vi "SDO_DRIVE_BEGIN.vi"(8 "error in (no error)":errorcluster) -> (0 "error out":errorcluster, 2 "Gyro Reading":T1 {"SIN" format="%13.4f"; "COS" format="%13.4f"; "VALUE" format="%13.4f"}, 3 "SWERVE_DRIVE_KINEMATICS":T2 {"SavedModuleStates"."Angle"."SIN" format="%13.4f"; "SavedModuleStates"."Angle"."COS" format="%13.4f"; "SavedModuleStates"."Angle"."VALUE" format="%13.4f"; "PrevCoR"."Y" format="%14.3f"; "PrevCoR"."X" format="%14.3f"; "Modules"."Y" format="%14.3f"; "Modules"."X" format="%14.3f"})   [LabVIEW 2019]
uses:
  <vilib>/Rock Robotics/WPI/ThirdParty/JAS_Junk/TrajLib/TypeDef/SWERVE_DRIVE_KINEMATICS.ctl
  <vilib>/Analysis/Matrix/Datatypes/RealMatrix.ctl
  <vilib>/Rock Robotics/WPI/ThirdParty/JAS_Junk/TrajLib/TypeDef/TRANSLATION2D.ctl
  <vilib>/Rock Robotics/WPI/ThirdParty/JAS_Junk/TrajLib/TypeDef/SWERVE_DRIVE_MODULE_STATE.ctl
  <vilib>/Rock Robotics/WPI/ThirdParty/JAS_Junk/TrajLib/TypeDef/ROTATION2D.ctl
  <vilib>/Rock Robotics/SystemInterfaces/DIO/FPGA_DIOPWMChannel.ctl
  <vilib>/Rock Robotics/SystemInterfaces/DIO/FPGA_DIOChannel.ctl
  <vilib>/Rock Robotics/SystemInterfaces/AI/FPGA_AIGyroChannel.ctl
  <vilib>/Rock Robotics/WPI/ThirdParty/JAS_Junk/TrajLib/Conv_Deg_Radians.vi
  <vilib>/Rock Robotics/WPI/ThirdParty/JAS_Junk/TrajLib/Rotation2d_CreateAngle.vi
  <vilib>/Rock Robotics/WPI/ThirdParty/JAS_Junk/TrajLib/VI/BoolCmd_Send_Internal.vi
  <vilib>/Rock Robotics/WPI/ThirdParty/JAS_Junk/TrajLib/VI/BoolCmd_ObtainQueue.vi
  SDO_DRIVE_GLOBALS.vi
  <vilib>/Rock Robotics/WPI/ThirdParty/JAS_Junk/TrajLib/Trajectory_Library.lvlib
  <vilib>/Rock Robotics/SystemInterfaces/AI/FPGA_AIChannel.ctl
  <vilib>/Rock Robotics/SystemInterfaces/spilib/spi_bus.ctl
  <vilib>/Rock Robotics/WPI/Gyro/WPI_GyroDevRef.ctl
  <vilib>/Analysis/Matrix/NI_Matrix.lvlib
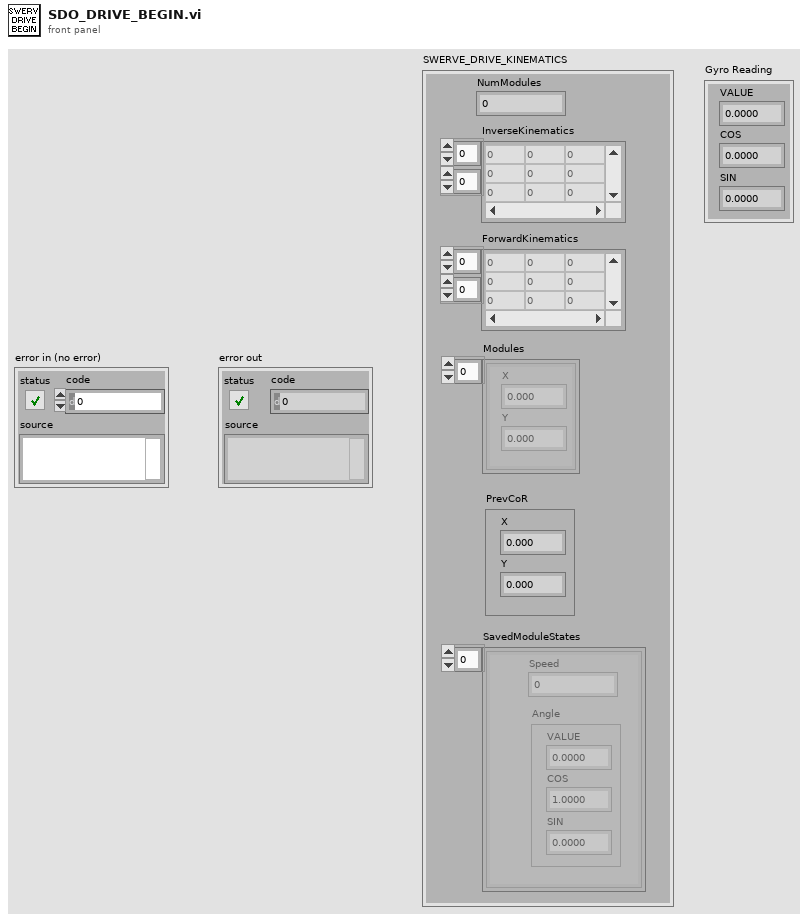
[diagram p1: front panel]
types:
  T1 = typedef "Trajectory_Library.lvlib/ROTATION2D.ctl" = cluster{"VALUE":dbl, "COS":dbl, "SIN":dbl}
  T2 = typedef "Trajectory_Library.lvlib/SWERVE_DRIVE_KINEMATICS.ctl" = cluster{"NumModules":i32, "InverseKinematics":T3, "ForwardKinematics":T3, "Modules":T4[], "PrevCoR":T4, "SavedModuleStates":T5[]}
  T3 = typedef "NI_Matrix.lvlib/RealMatrix.ctl" = dbl[][]
  T4 = typedef "Trajectory_Library.lvlib/TRANSLATION2D.ctl" = cluster{"X":dbl, "Y":dbl}
  T5 = typedef "Trajectory_Library.lvlib/SWERVE_DRIVE_MODULE_STATE.ctl" = cluster{"Speed":dbl, "Angle":T1}
  T6 = typedef "FPGA_AIGyroChannel.ctl" = enum8{"AI 0", "AI 1", "Invalid"}
  T7 = typedef "FPGA_DIOChannel.ctl" = enum8{"DIO 0", "DIO 1", "DIO 2", "DIO 3", "DIO 4", "DIO 5", "DIO 6", "DIO 7", "DIO 8", "DIO 9", "DIO MXP 0", "DIO MXP 1", "DIO MXP 2", "DIO MXP 3", "DIO MXP 4", "DIO MXP 5", "DIO MXP 6", "DIO MXP 7", "DIO MXP 8", "DIO MXP 9", "DIO MXP 10", "DIO MXP 11", "DIO MXP 12", "DIO MXP 13", "DIO MXP 14", "DIO MXP 15", "SPI Port CS1", "SPI Port CS2", "SPI Port CS3", "SPI Port MISO", "SPI Port MOSI", "Invalid"}
  T8 = typedef "FPGA_DIOPWMChannel.ctl" = enum8{"PWM 0", "PWM 1", "PWM 2", "PWM 3", "PWM 4", "PWM 5", "PWM 6", "PWM 7", "PWM 8", "PWM 9", "PWM MXP 0", "PWM MXP 1", "PWM MXP 2", "PWM MXP 3", "PWM MXP 4", "PWM MXP 5", "PWM MXP 6", "PWM MXP 7", "PWM MXP 8", "PWM MXP 9", "Invalid"}
  T9 = typedef "WPI_GyroDevRef.ctl" = cluster{"DevStatus":errorcluster, "Analog Channel":T10, "Gain (VoltsPerDegree/Second)":dbl, "Gyro Type":enum16{"Analog", "XRS450"}, "Handle":i32, "SPI Bus":T11, "Device Found":bool, "Sample Rate":dbl, "Calibrate On Open":bool, "Offset":dbl}
  T10 = typedef "FPGA_AIChannel.ctl" = enum8{"AI 0", "AI 1", "AI 2", "AI 3", "AI MXP 0", "AI MXP 1", "AI MXP 2", "AI MXP 3", "Invalid"}
  T11 = typedef "spi_bus.ctl" = enum16{"SPI On-Board, CS0", "SPI On-Board, CS1", "SPI On-Board, CS2", "SPI On-Board, CS3", "SPI MXP", "Invalid"}
  T12 = typedef "Trajectory_Library.lvlib/SWERVE_DRIVE_MODULE_POSITION.ctl" = cluster{"Distance":dbl, "Angle":T1, "P":bool}
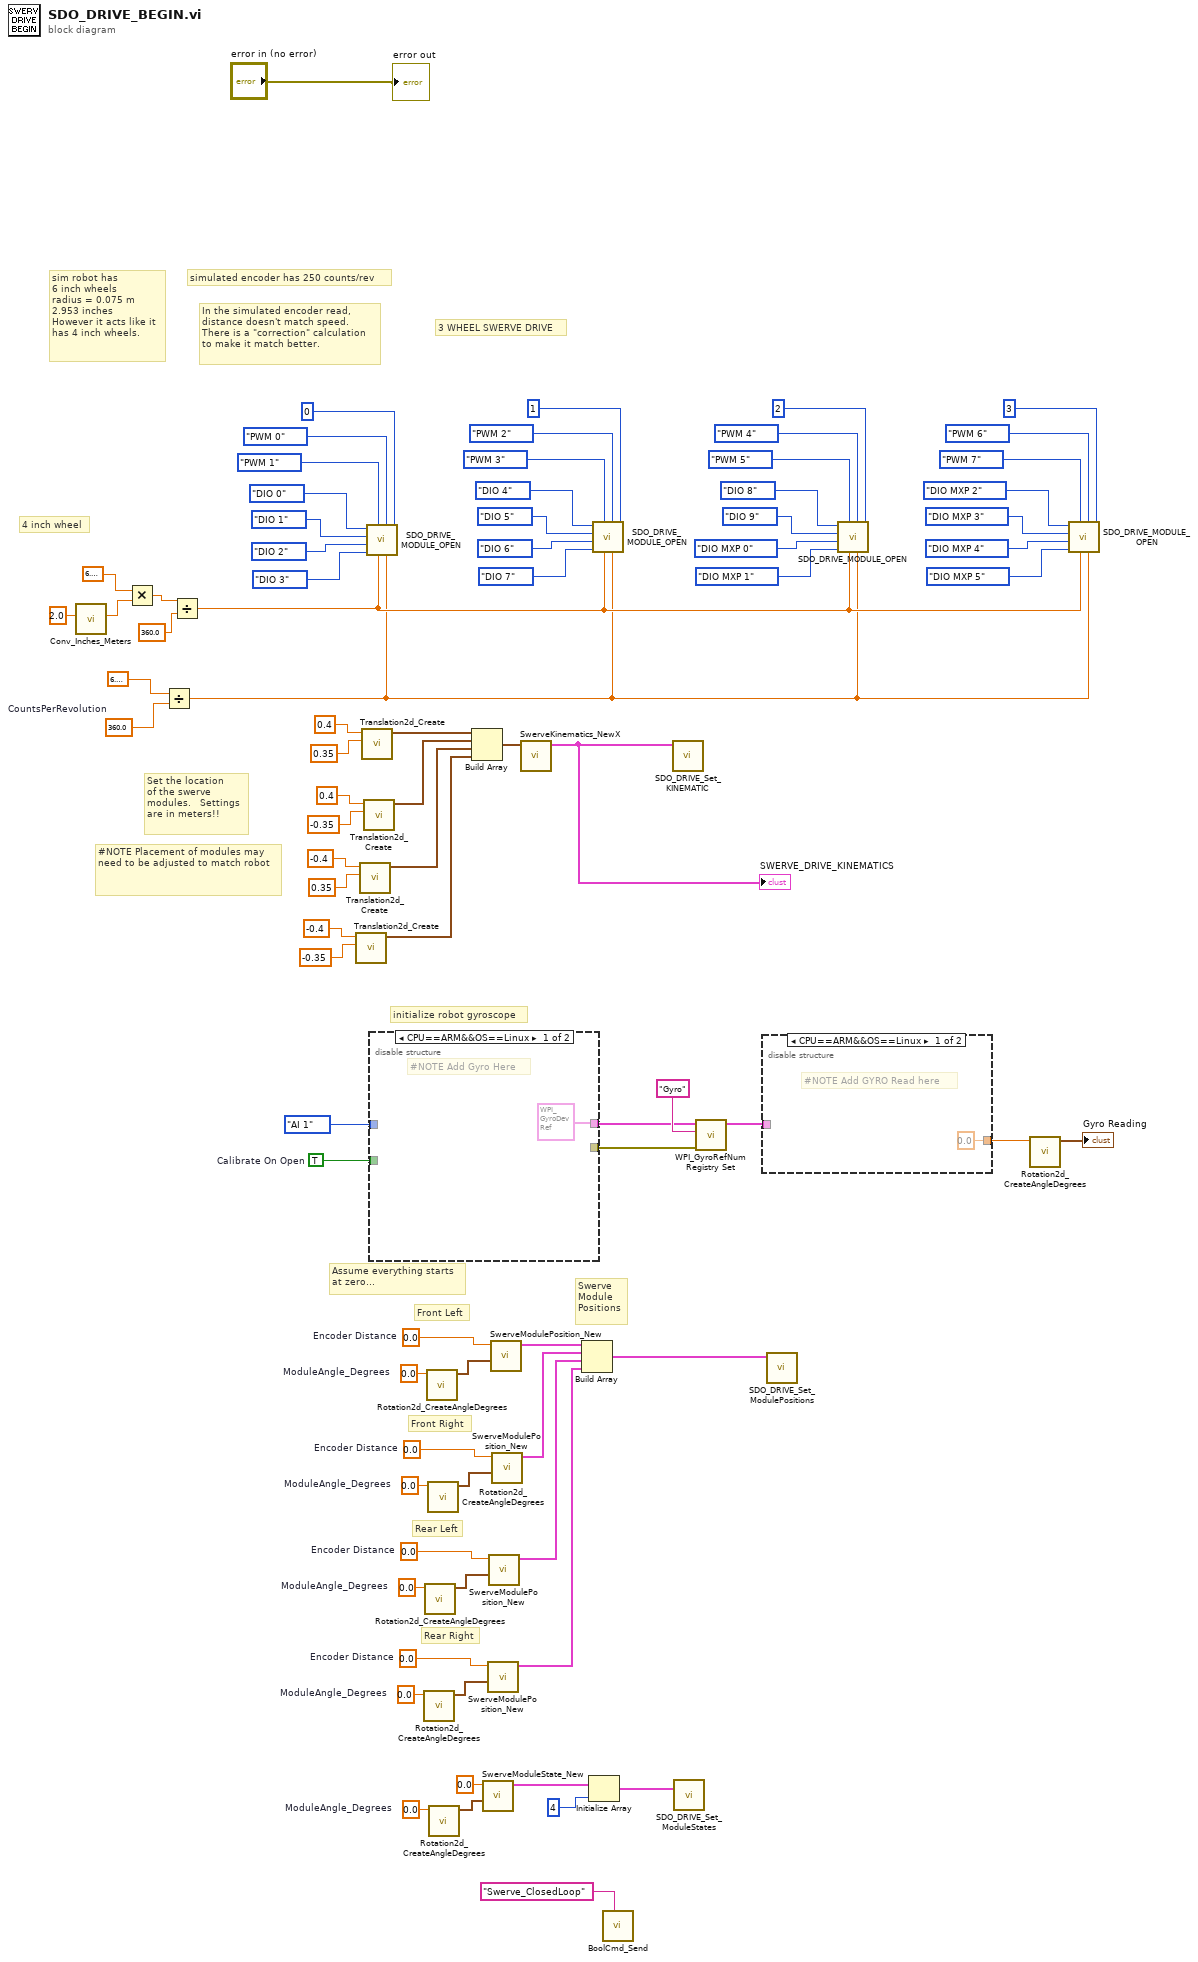
[diagram p0: block diagram]
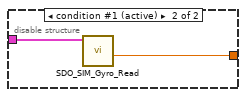
[diagram p2: hidden frame]
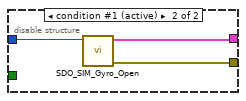
[diagram p3: hidden frame]
diagram:
  w6 = 0.0  # ModuleAngle_Degrees
  w29 = 0.0  # ModuleAngle_Degrees
  w27 = 0.0  # Encoder Distance
  w26 = 0.0  # ModuleAngle_Degrees
  w24 = 0.0  # Encoder Distance
  w23 = 0.0  # ModuleAngle_Degrees
  w21 = 0.0  # Encoder Distance
  w19 = 0.0  # ModuleAngle_Degrees
  w17 = 0.0  # Encoder Distance
  w46 = 360.0  # CountsPerRevolution
  w15 = TRUE  # Calibrate On Open
  # "Assume everything starts\nat zero..."
  # "Front Left"
  # "Swerve\nModule\nPositions"
  # "Rear Right"
  # "Rear Left"
  # "Front Right"
  # "#NOTE Placement of modules may need to be adjusted to match robot"
  # "Set the location\nof the swerve \nmodules.   Settings\nare in meters!!"
  # "4 inch wheel"
  # "3 WHEEL SWERVE DRIVE"
  # "initialize robot gyroscope"
  # "In the simulated encoder read,\ndistance doesn't match speed.\nThere is a \"correction\" calculation\nto make it match better."
  # "simulated encoder has 250 counts/rev"
  # "sim robot has\n6 inch wheels\nradius = 0.075 m\n2.953 inches\nHowever it acts like it\nhas 4 inch wheels."
  n1 = call <vilib>:"Conv_Inches_Meters.vi"("INCH"=2.0) -> ("Meters"=w71:dbl)  [unwired: 10 in]
  n2 = Multiply(x=6.283185307179586, y=w71) -> (x*y=w34:dbl)
  n3 = Divide(x=6.283185307179586, y=w46) -> (x/y=w80:dbl)
  n4 = Divide(x=w34, y=360.0) -> (x/y=w81:dbl)
  n5 = call <vilib>:"Translation2d_Create.vi"("Y"=-0.35, "X"=-0.4) -> ("TRANSLATION"=w84:T4)  [unwired: 9 in]
  n6 = call <vilib>:"Translation2d_Create.vi"("Y"=0.35, "X"=-0.4) -> ("TRANSLATION"=w69:T4)  [unwired: 9 in]
  n7 = call <vilib>:"Translation2d_Create.vi"("Y"=0.35, "X"=0.4) -> ("TRANSLATION"=w67:T4)  [unwired: 9 in]
  n8 = call <vilib>:"Translation2d_Create.vi"("Y"=-0.35, "X"=0.4) -> ("TRANSLATION"=w68:T4)  [unwired: 9 in]
  n9 = call "SDO_DRIVE_MODULE_OPEN.vi"("Module Index"=0 ("NameSuffix"), "RadiansPerCount"=w80, "Drive PWM Channel"=FPGA_DIOPWMChannel."PWM 0", "DistancePerCount"=w81, "Swerve PWM Channel"=FPGA_DIOPWMChannel."PWM 1", "Swerve B Channel"=FPGA_DIOChannel."DIO 3", "Swerver A Channel"=FPGA_DIOChannel."DIO 2", "Drive B Channel"=FPGA_DIOChannel."DIO 1", "Drive A channel"=FPGA_DIOChannel."DIO 0") -> ()  [unwired: 3 in]
  n10 = disable-structure shown="CPU==ARM&&OS==Linux" {
    disable-tunnel: w15 -> [_ _]
    disable-tunnel: [T9 {"DevStatus"={"status"=FALSE, "code"=0, "source"=""}, "Analog Channel"=enum."AI 1", "Gain (VoltsPerDegree/Second)"=0.0, "Gyro Type"=enum."Analog", "Handle"=0, "SPI Bus"=enum."Invalid", "Device Found"=FALSE, "Sample Rate"=1.0, "Calibrate On Open"=FALSE, "Offset"=0.0} ("GyroDevRef") w88] -> w14
    disable-tunnel: [_ w87] -> w13
    disable-tunnel: FPGA_AIGyroChannel."AI 1" ("Analog Channel") -> [_ w86]
    frame condition #0 {
      # "#NOTE Add Gyro Here"
    }
    frame condition #1 (active) {
      n11 = call "SDO_SIM_Gyro_Open.vi"("Analog Channel"=w86) -> ("error out"=w87:errorcluster, "GyroDevRef"=w88:T9)  [unwired: 9 in]
    }
  }
  n12 = call <vilib>:"Rotation2d_CreateAngleDegrees.vi"("Angle_Degrees"=w29) -> ("ROTATION"=w28:T1)  [unwired: 10 in]
  n13 = call <vilib>:"Rotation2d_CreateAngleDegrees.vi"("Angle_Degrees"=w26) -> ("ROTATION"=w25:T1)  [unwired: 10 in]
  n14 = call <vilib>:"Rotation2d_CreateAngleDegrees.vi"("Angle_Degrees"=w19) -> ("ROTATION"=w18:T1)  [unwired: 10 in]
  n15 = call <vilib>:"Rotation2d_CreateAngleDegrees.vi"("Angle_Degrees"=w23) -> ("ROTATION"=w22:T1)  [unwired: 10 in]
  n16 = call <vilib>:"Rotation2d_CreateAngleDegrees.vi"("Angle_Degrees"=w6) -> ("ROTATION"=w5:T1)  [unwired: 10 in]
  n17 = Build Array(w67, w68, w69, w84) -> (w70:T4[])
  n18 = call <vilib>:"SwerveModuleState_New.vi"("ROTATION"=w5, "Speed"=0.0) -> ("SWERVE_DRIVE_MODULE_STATE"=w4:T5)  [unwired: 9 in]
  n19 = call <vilib>:"SwerveModulePosition_New.vi"("ROTATION"=w28, "Distance"=w27) -> ("SWERVE_DRIVE_MODULE_POSITION"=w32:T12)  [unwired: 9 in]
  n20 = call <vilib>:"SwerveModulePosition_New.vi"("ROTATION"=w25, "Distance"=w24) -> ("SWERVE_DRIVE_MODULE_POSITION"=w31:T12)  [unwired: 9 in]
  n21 = call <vilib>:"SwerveModulePosition_New.vi"("ROTATION"=w18, "Distance"=w17) -> ("SWERVE_DRIVE_MODULE_POSITION"=w20:T12)  [unwired: 9 in]
  n22 = call <vilib>:"SwerveModulePosition_New.vi"("ROTATION"=w22, "Distance"=w21) -> ("SWERVE_DRIVE_MODULE_POSITION"=w30:T12)  [unwired: 9 in]
  n23 = call <vilib>:"SwerveKinematics_NewX.vi"("Wheels"=w70) -> ("SWERVE_DRIVE_KINEMATICS"=w2:T2)  [unwired: 10 in]
  "SWERVE_DRIVE_KINEMATICS" <- w2
  n24 = Build Array(w20, w30, w31, w32) -> (w3:T12[])
  n25 = Initialize Array(w4, 4 ("dimension size")) -> (w1:T5[])
  n26 = call "SDO_DRIVE_MODULE_OPEN.vi"("Module Index"=1 ("NameSuffix"), "RadiansPerCount"=w80, "Drive PWM Channel"=FPGA_DIOPWMChannel."PWM 2", "DistancePerCount"=w81, "Swerve PWM Channel"=FPGA_DIOPWMChannel."PWM 3", "Swerve B Channel"=FPGA_DIOChannel."DIO 7", "Swerver A Channel"=FPGA_DIOChannel."DIO 6", "Drive B Channel"=FPGA_DIOChannel."DIO 5", "Drive A channel"=FPGA_DIOChannel."DIO 4") -> ()  [unwired: 3 in]
  n27 = call <vilib>:"BoolCmd_Send.vi"("Command Name"="Swerve_ClosedLoop") -> ()  [unwired: 10 in, 1 out]
  n28 = call "SDO_DRIVE_Set_KINEMATIC.vi"("SWERVE_DRIVE_KINEMATICS"=w2) -> ()  [unwired: 11 in]
  n29 = call "SDO_DRIVE_Set_ModuleStates.vi"("Swerve Module States"=w1) -> ()  [unwired: 11 in]
  n30 = call <vilib>:"WPI_GyroRefNum Registry Set.vi"("error in (no error)"=w13, "refnum name"="Gyro", "GyroDevRef"=w14) -> ("GyroDevRef"=w11:T9)  [unwired: 7 in, 1 out]
  n31 = disable-structure shown="CPU==ARM&&OS==Linux" {
    disable-tunnel: w11 -> [_ w91]
    disable-tunnel: [0.0 ("Gyro_Cont_Deg") w90] -> w10
    frame condition #0 {
      # "#NOTE Add GYRO Read here"
    }
    frame condition #1 (active) {
      n32 = call "SDO_SIM_Gyro_Read.vi"("GyroDevRef"=w91) -> ("Gyro_Cont_Deg"=w90:dbl)  [unwired: 10 in]
    }
  }
  n33 = call "SDO_DRIVE_Set_ModulePositions.vi"("Swerve Module Positions"=w3) -> ()  [unwired: 11 in]
  n34 = call "SDO_DRIVE_MODULE_OPEN.vi"("Module Index"=2 ("NameSuffix"), "RadiansPerCount"=w80, "Drive PWM Channel"=FPGA_DIOPWMChannel."PWM 4", "DistancePerCount"=w81, "Swerve PWM Channel"=FPGA_DIOPWMChannel."PWM 5", "Swerve B Channel"=FPGA_DIOChannel."DIO MXP 1", "Swerver A Channel"=FPGA_DIOChannel."DIO MXP 0", "Drive B Channel"=FPGA_DIOChannel."DIO 9", "Drive A channel"=FPGA_DIOChannel."DIO 8") -> ()  [unwired: 3 in]
  n35 = call <vilib>:"Rotation2d_CreateAngleDegrees.vi"("Angle_Degrees"=w10) -> ("ROTATION"=→"Gyro Reading":T1)  [unwired: 10 in]
  n36 = call "SDO_DRIVE_MODULE_OPEN.vi"("Module Index"=3 ("NameSuffix"), "RadiansPerCount"=w80, "Drive PWM Channel"=FPGA_DIOPWMChannel."PWM 6", "DistancePerCount"=w81, "Swerve PWM Channel"=FPGA_DIOPWMChannel."PWM 7", "Swerve B Channel"=FPGA_DIOChannel."DIO MXP 5", "Swerver A Channel"=FPGA_DIOChannel."DIO MXP 4", "Drive B Channel"=FPGA_DIOChannel."DIO MXP 3", "Drive A channel"=FPGA_DIOChannel."DIO MXP 2") -> ()  [unwired: 3 in]
  "error out" <- "error in (no error)"
